vi "Delete Active DUT Connector.vi"(8 "error in (no error)":errorcluster, 10 "Connector (\"Connector1\")":string="Connector1", 11 "VISA resource name":refnum<visa-resource-name>) -> (0 "error out":errorcluster, 3 "VISA resource name out":refnum<visa-resource-name>)   [LabVIEW 2020, in "Rohde&Schwarz CMXP Base.lvlib"]
doc: "Deletes an antenna connector of the active DUT.\n\nAttribute:\nRSCMXPBASE_ATTR_ACTIVE_DUT_CONNECTOR_DELETE\n\nRemote-control command:\nDELete:DUT:CONNector"
uses:
  <instrlib>/Rohde&Schwarz CMXP Base/Rohde&Schwarz CMXP Base.lvlib
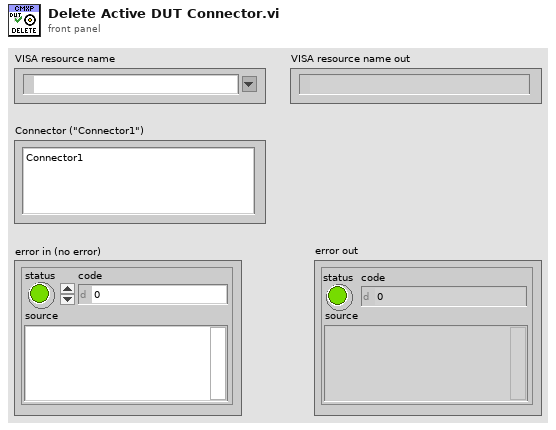
[diagram p1: front panel]
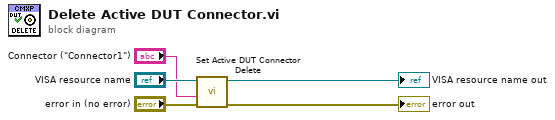
[diagram p0: block diagram]
diagram:
  n1 = call "Set Active DUT Connector Delete"("error in (no error)"="error in (no error)", "Active DUT Connector Delete ()"="Connector (\"Connector1\")", "instrument handle"="VISA resource name") -> ("error out"=→"error out":errorcluster, "instrument handle out"=→"VISA resource name out":refnum<visa-resource-name>)  [unwired: 7 in]
